vi "RT_Main.vi"() -> ()   [LabVIEW 2019]
uses:
  <vilib>/Platform/TimedLoop/XDataNode/timing_clust.ctl
  <vilib>/Platform/TimedLoop/XDataNode/nitl_modes.ctl
  <vilib>/Platform/TimedLoop/XDataNode/wakeup.ctl
  <vilib>/FPGAPlugInAG/myRIO-1900/niLvFpga_Open_myRIO-1900.vi
  <vilib>/rvi/interface/common/dynamic/niFpgaDynamicAddResources.vi
  <vilib>/Utility/error.llb/Error Cluster From Error Code.vi
  <vilib>/rvi/errors/niLvFpgaAdjustHostInterfaceError.vi
  <vilib>/rvi/interface/common/niFpgaWaitOnOcc.vi
  <vilib>/FPGAPlugInAG/Dynamic/niLvFpga_Run_Dynamic.vi
  <vilib>/FPGAPlugInAG/Dynamic/niLvFpga_Close_Dynamic.vi
  <vilib>/rvi/interface/nirviOpenFPGA/nirviOpenFPGA.xnode
  FPGA Bitfiles/lab4_FPGATarget2_FPGAmain_rUDf5eu67Sc.lvbitx
  FPGA_main.vi
  <vilib>/rvi/interface/nirviReadWriteControl/nirviReadWriteControl.xnode
  <vilib>/rvi/interface/nirviMethod/nirviMethod.xnode
  <vilib>/platform/TimedLoop/XDataNode/XDataNode.xnode
  <vilib>/rvi/interface/nirviCloseFPGA/nirviCloseFPGA.xnode
  <vilib>/rvi/interface/Simulation/niFpgaSimulationCallBeginRW.vi
  <vilib>/rvi/errors/niLvFpgaMergeErrorWithErrorCode.vi
  <vilib>/FPGAPlugInAG/Dynamic/niLvFpga_ReadFifo_Dynamic.vi
  <vilib>/Platform/TimedLoop/XDataNode/XDNodeRunTimeDep.lvlib
  NiFpgaLv.dll
  <vilib>/FPGAPlugInAG/Dynamic/niLvFpga_ConfigureFifo_Dynamic.vi
  <vilib>/FPGAPlugInAG/Dynamic/niLvFpga_StartFifo_Dynamic.vi
panel:
  out "Data Recieved":i32
  out "Waveform Graph":i16[][](graph)
  in  "Monitoring?":bool
  in  "TriggerLevelZ":i16
  in  "TriggerLevelY":i16
  in  "TriggerLevelX":i16
  in  "stop":bool
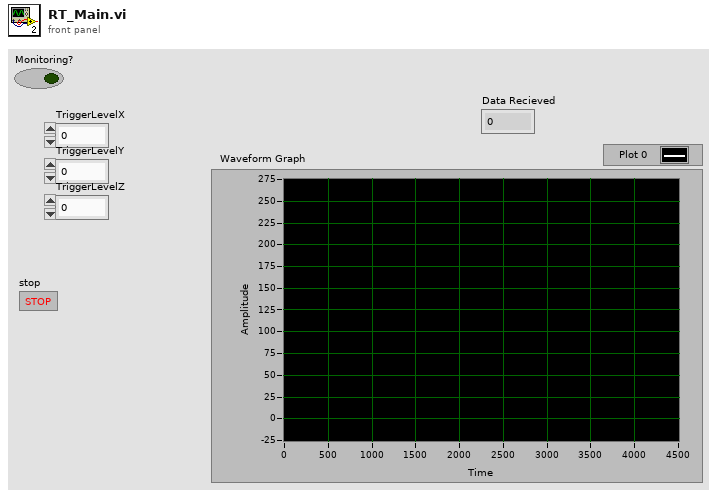
[diagram p1: front panel]
types:
  T1 = typedef "XDNodeRunTimeDep.lvlib/timing_clust.ctl" = cluster{"Expected End [f-1]":u64, "Actual End [f-1]":u64, "Finished Late? [f-1]":bool, "Expected End [i-1]":u64, "Actual End [i-1]":u64, "Finished Late? [i-1]":bool, "Expected Start [i]":u64, "Actual Start [i]":u64, "Expected Start [f]":u64, "Actual Start [f]":u64, "Source Name":string, "Structure Name":string, "Period":i64, "Deadline":i64, "Offset":i64, "Start":i64, "Priority":i32, "Timeout":i32, "Mode":T2, "Wakeup Reason":T3, "Error":errorcluster, "Source Type":string, "Secondary Source Type":string, "Global End Time":u64, "Global Start Time":u64, "Frame Duration":u64, "Iteration Duration":u64, "Assigned CPU":i32, "I/O Scan Engine Mode":u32}
  T2 = typedef "XDNodeRunTimeDep.lvlib/nitl_modes.ctl" = enum32{"No Change", "Process missed periods, maintain original phase", "Discard missed periods, maintain original phase", "Process missed periods, ignore original phase", "Discard missed periods, ignore original phase"}
  T3 = typedef "XDNodeRunTimeDep.lvlib/wakeup.ctl" = enum32{"Normal", "Aborted", "Asynchronous wakeup", "Timing source error", "Timed loop error", "Timeout"}
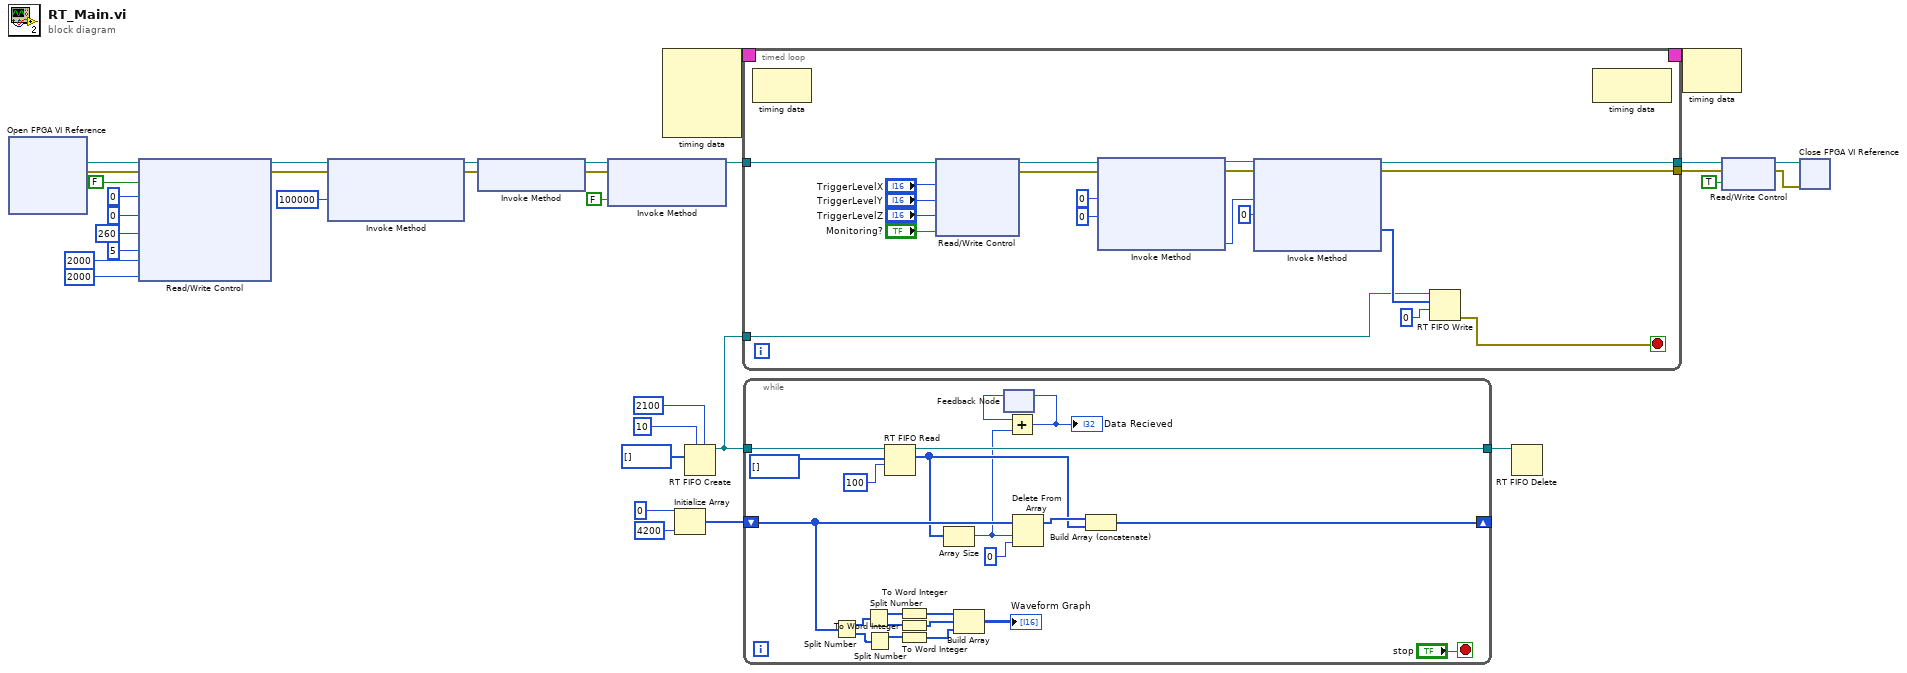
[diagram p0: block diagram]
diagram:
  n1 = xnode "Open FPGA VI Reference"() -> ("FPGA VI Reference Out"=w33:refnum<k20>, "error out"=w23:errorcluster)  [unwired: 2 in]
  n2 = xnode "Read/Write Control"("FPGA VI Reference In"=w33, "error in"=w23, "stop"=FALSE, "TriggerX"=i16 0, "TriggerY"=i16 0, "TriggerZ"=i16 260, "SamplesOverTreshold"=u8 5, "PretriggerLenght"=u16 2000, "PosttriggerLenght"=u16 2000) -> ("FPGA VI Reference Out"=w27:refnum<k20>, "error out"=w22:errorcluster)
  n3 = xnode "Invoke Method"("FPGA VI Reference In"=w27, "error in"=w22, "Requested Depth"=u32 100000) -> ("FPGA VI Reference Out"=w25:refnum<k20>, "error out"=w21:errorcluster)  [unwired: 1 out]
  n4 = xnode "Invoke Method"("FPGA VI Reference In"=w25, "error in"=w21) -> ("FPGA VI Reference Out"=w24:refnum<k20>, "error out"=w20:errorcluster)
  n5 = xnode "Invoke Method"("FPGA VI Reference In"=w24, "error in"=w20, "Wait Until Done (F)"=FALSE) -> ("FPGA VI Reference Out"=w19:refnum<k20>)  [unwired: 1 out]
  n6 = node-c288() -> (w18:T1)  [unwired: 4 in]
  n7 = Initialize Array(u64 0 ("element"), 4200 ("dimension size")) -> (w2:u64[])
  n8 = RT FIFO Create(1:u64[] [] ("Data"), 4:u32 10 ("size (10)"), 6:u32 2100 ("elements in array (1)")) -> (8:w5:refnum<k33>)  [unwired: 5 in, 2 out]
  n9 = timed-loop {
    timing: w18 -> [_]
    timing-out: [_] -> w17
    tunnel: w19 -> [w52]
    tunnel: [w51] -> w16
    tunnel: [w50] -> w12
    tunnel: w5 -> [w36]
    stop <- w34 stop-if-true
    n10 = node-c288() -> ()  [unwired: 1 in, 1 out]
    n11 = xnode "Read/Write Control"("FPGA VI Reference In"=w52, "TriggerX"="TriggerLevelX", "TriggerY"="TriggerLevelY", "TriggerZ"="TriggerLevelZ", "Monitoring?"="Monitoring?") -> ("FPGA VI Reference Out"=w46:refnum<k20>, "error out"=w44:errorcluster)  [unwired: 1 in]
    n12 = xnode "Invoke Method"("FPGA VI Reference In"=w46, "error in"=w44, "Number of Elements"=u32 0, "Timeout (ms)"=0) -> ("FPGA VI Reference Out"=w45:refnum<k20>, "error out"=w43:errorcluster, "Elements Remaining"=w40:u32)  [unwired: 1 out]
    n13 = xnode "Invoke Method"("FPGA VI Reference In"=w45, "error in"=w43, "Number of Elements"=w40, "Timeout (ms)"=0) -> ("FPGA VI Reference Out"=w51:refnum<k20>, "error out"=w50:errorcluster, "Data"=w37:u64[])  [unwired: 1 out]
    n14 = RT FIFO Write(0:w36, 1:w37, 2:0 ("timeout in ms (0)")) -> (11:w34:errorcluster)  [unwired: 2 in, 3 out]
    n15 = node-c288() -> ()  [unwired: 1 in, 1 out]
  }
  n16 = while {
    tunnel: w5 -> [w76]
    tunnel: [w59] -> w6
    shift-right: [w58] -> _
    shift-left: w2 -> [w62]
    stop <- "stop" stop-if-true
    n17 = Split Number(x=w62) -> (hi(x)=w71:u32[], lo(x)=w64:u32[])
    n18 = Split Number(x=w71) -> (hi(x)=w70:u16[], lo(x)=w68:u16[])
    n19 = Split Number(x=w64) -> (hi(x)=w69:u16[])  [unwired: 1 out]
    n20 = RT FIFO Read(0:w76, 1:u64[] [] ("element"), 2:100 ("timeout in ms (0)")) -> (8:w59:refnum<k33>, 9:w60:u64[])  [unwired: 1 in, 3 out]
    n21 = To Word Integer(number=w70) -> (16bit integer=w67:i16[])
    n22 = To Word Integer(number=w68) -> (16bit integer=w66:i16[])
    n23 = To Word Integer(number=w69) -> (16bit integer=w65:i16[])
    n24 = Array Size(array=w60) -> (size(s)=w57:i32)
    n25 = Build Array(w67, w66, w65) -> (→"Waveform Graph":i16[][])
    n26 = feedback #1() -> (w55:i32)  [unwired: 1 in]
    n27 = Add(x=w55, y=w57) -> (x+y=w56:i32)
    "Data Recieved" <- w56
    n28 = feedback-in #1(w56) -> ()
    n29 = Delete From Array(array=w62, length=w57, index=0) -> (array with subset deleted=w72:u64[])  [unwired: 1 out]
    n30 = Build Array (concatenate)(w72, w60) -> (w58:u64[])
  }
  n31 = RT FIFO Delete(0:w6) -> ()  [unwired: 2 in, 1 out]
  n32 = node-c288(w17) -> ()  [unwired: 1 out]
  n33 = xnode "Read/Write Control"("FPGA VI Reference In"=w16, "error in"=w12, "stop"=TRUE) -> ("FPGA VI Reference Out"=w14:refnum<k20>, "error out"=w13:errorcluster)
  n34 = xnode "Close FPGA VI Reference"("FPGA VI Reference In"=w14, "error in"=w13) -> ()  [unwired: 1 out]
